vi "MaxX.vi"() -> ()   [LabVIEW 2010]
panel:
  in  "X Max in":u32=1 min=1 step=1
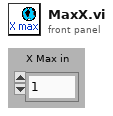
[diagram p1: front panel]
diagram:
